vi "GUI.vi"(8 "error in (no error)":errorcluster) -> (0 "error out":errorcluster)   [LabVIEW 2017]
uses:
  Type Definitions/Queue FG Options.ctl
panel:
  in  "Transactions":T1
  out "Pinpad":T2
  in  "Card Reader":bool
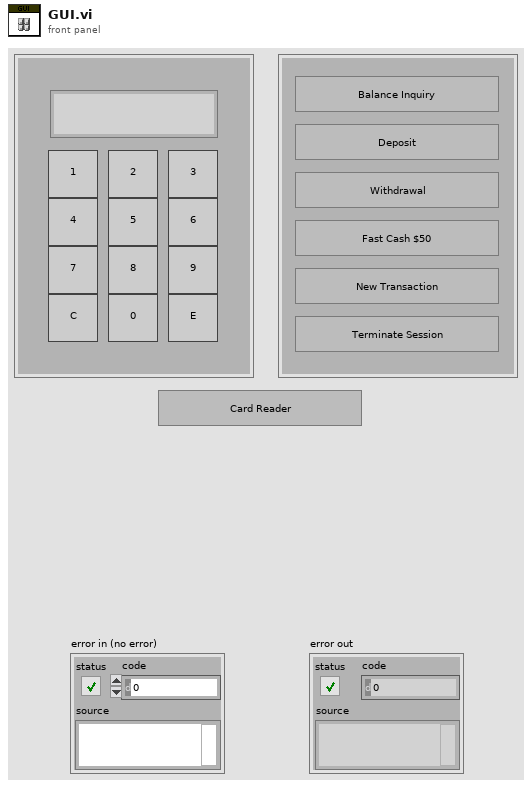
[diagram p1: front panel]
types:
  T1 = cluster{"Balance Inquiry":bool, "Deposit":bool, "Withdrawal":bool, "Fast Cash $50":bool, "New Transaction":bool, "Terminate Session":bool}
  T2 = cluster{"Screen":string, "num1":bool, "num2":bool, "num3":bool, "num6":bool, "num5":bool, "num4":bool, "num7":bool, "num8":bool, "num9":bool, "C":bool, "num0":bool, "E":bool}
  T3 = typedef "Queue FG Options.ctl" = enum16{"Set", "Get", "Read", "Write"}
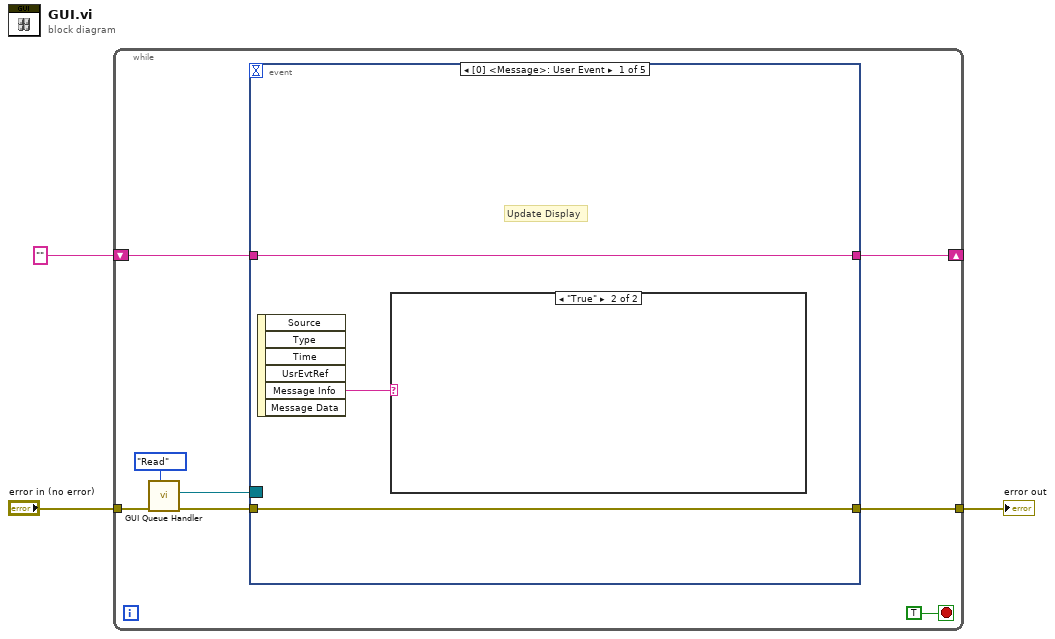
[diagram p0: block diagram]
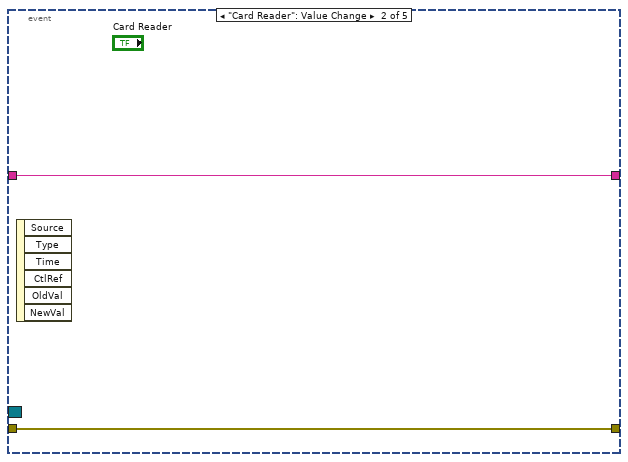
[diagram p3: hidden frame]
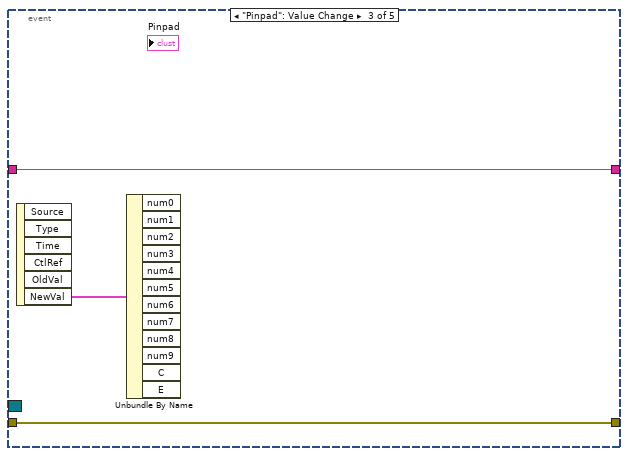
[diagram p4: hidden frame]
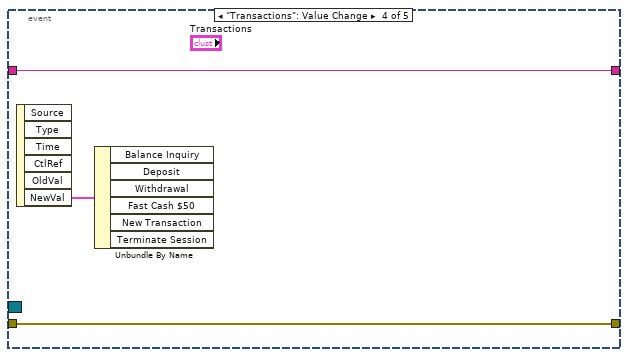
[diagram p5: hidden frame]
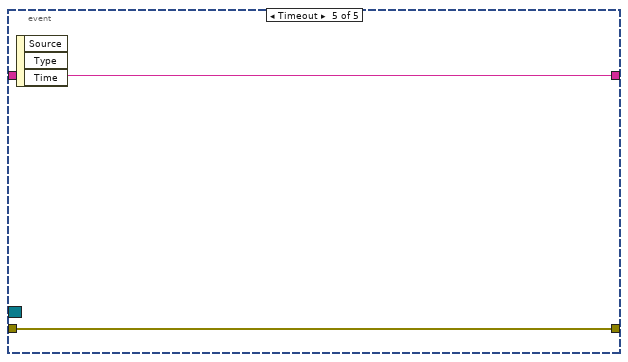
[diagram p6: hidden frame]
diagram:
  n1 = while {
    tunnel: "error in (no error)" -> [w10]
    tunnel: [w7] -> w2
    shift-right: [w4] -> _
    shift-left: "" -> [w5]
    stop <- TRUE stop-if-true
    n2 = call "GUI Queue Handler.vi"("Action"=Queue_FG_Options."Read", "error in (no error)"=w10) -> ("error out"=w8:errorcluster, "Event Registration Refnum out"=w6:refnum<event-registration>)  [unwired: 7 in, 1 out]
    n3 = event shown="[0] <Message>: User Event" {
      selector: w6 -> [_ _ _ _ _]
      dyn-events: _ -> [_ _ _ _ _]
      timeout: _ -> [_ _ _ _ _]
      tunnel: w8 -> [w13 w15 w17 w20 w24]
      tunnel: [w13 w15 w17 w20 w24] -> w7
      tunnel: w5 -> [w14 w16 w18 w21 w23]
      tunnel: [w14 w16 w18 w21 w23] -> w4
      event User Event {
        # "Update Display"
        n4 = event-data() -> ("Message Info"=w12:string)  [unwired: 1 in, 5 out]
        n5 = case shown="\"True\"" w12 {
          frame "False", Default {
          }
          frame "True" {
          }
        }
      }
      event "Card Reader": Value Change {
        n6 = event-data() -> ()  [unwired: 1 in, 6 out]
      }
      event "Pinpad": Value Change {
        n7 = event-data() -> ("NewVal"=w19:T2)  [unwired: 1 in, 5 out]
        n8 = Unbundle By Name(w19) -> ()  [unwired: 12 out]
      }
      event "Transactions": Value Change {
        n9 = event-data() -> ("NewVal"=w22:T1)  [unwired: 1 in, 5 out]
        n10 = Unbundle By Name(w22) -> ()  [unwired: 6 out]
      }
      event Timeout {
        n11 = event-data() -> ()  [unwired: 1 in, 3 out]
      }
    }
  }
  "error out" <- w2
